vi "Get ni-xnet port Info.vi"(8 "Error In":errorcluster, 11 "NI-XNET Port Item Ref in":T1 format="%.0x") -> (0 "Error Out":errorcluster, 1 "NI-XNET Port Type":string, 2 "NI-XNET Port Name":string, 3 "NI-XNET Port Item Ref out":T1 format="%.0x", 4 "NI-XNET Port Number":i32)   [LabVIEW 2018, in "NI-XNET Monitor System Explorer.lvlib"]
uses:
  NI-XNET Monitor System Explorer.lvlib
  <vilib>/NI Veristand/Custom Device API/Custom Device Item Ref.ctl
  <vilib>/NI Veristand/Custom Device API/Get Item Property (I32).vi
  <vilib>/NI VeriStand/Custom Device API/Custom Device API.lvlib
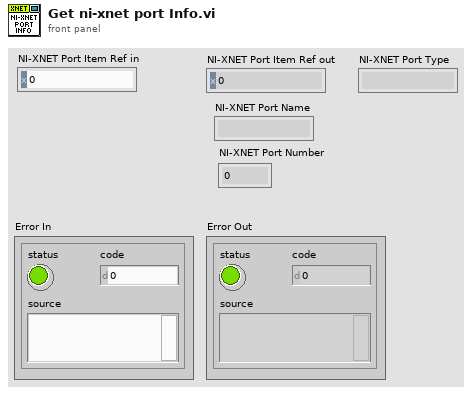
[diagram p1: front panel]
types:
  T1 = typedef "Custom Device API.lvlib/Custom Device Item Ref.ctl" = u64
  T2 = typedef "Custom Device API.lvlib/Custom Device Item Info.ctl" = cluster{"Name":string, "Is Channel":bool, "GUID":string, "Is Waveform":bool}
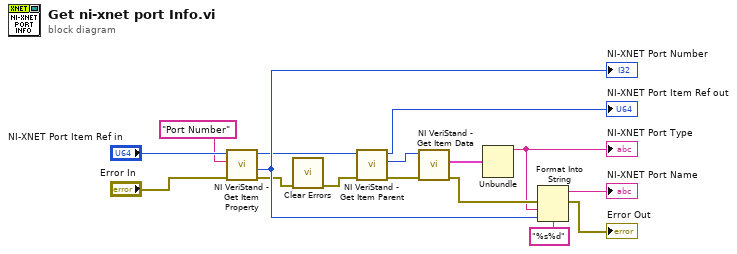
[diagram p0: block diagram]
diagram:
  n1 = call-poly <vilib>:"NI VeriStand - Get Item Property.vi"("error in (no error)"="Error In", "Property Name"="Port Number", "Item Ref in"="NI-XNET Port Item Ref in") -> ("error out"=w12:errorcluster, "Value"=w15:i32, "Item Ref out"=w14:T1)  [unwired: 5 in, 1 out]
  "NI-XNET Port Number" <- w15
  n2 = call <vilib>:"Clear Errors.vi"("error in (no error)"=w12) -> ("error out"=w5:errorcluster)  [unwired: 5 in, 1 out]
  n3 = call <vilib>:"NI VeriStand - Get Item Parent.vi"("error in (no error)"=w5, "Item Ref in"=w14) -> ("error out"=w9:errorcluster, "Parent Ref"=w4:T1, "Item Ref out"=→"NI-XNET Port Item Ref out":T1)  [unwired: 6 in, 1 out]
  n4 = call <vilib>:"NI VeriStand - Get Item Data.vi"("error in (no error)"=w9, "Item Ref in"=w4) -> ("error out"=w10:errorcluster, "Item Info"=w8:T2)  [unwired: 6 in, 2 out]
  n5 = Unbundle(w8) -> ("Name"=w3:string)  [unwired: 3 out]
  "NI-XNET Port Type" <- w3
  n6 = Format Into String(format string="%s%d", error in=w10, w3, w15) -> (resulting string=→"NI-XNET Port Name":string, error out=→"Error Out":errorcluster)  [unwired: 1 in]
